vi "openUMARov.vi"() -> ()   [LabVIEW 2019]
uses:
  <userlib>/ROS for LabVIEW Software/Examples/ROS Examples/Control 1.ctl
  <userlib>/ROS for LabVIEW Software/ROS/Code/Console/Servers/ServerSubs/TopicDef.ctl
  <userlib>/ROS for LabVIEW Software/ROS/Code/SubVIs/_ROSDirection.ctl
  <vilib>/event_ctls.llb/eventvkey.ctl
  <userlib>/ROS for LabVIEW Software/ROS/MessageParsing/std_msgs/subs/parse_float32_scalar.vi
  <userlib>/ROS for LabVIEW Software/ROS/MessageBuilding/std_msgs/subs/float32Scalar.vi
panel:
  in  "Size":string(combo)="mid"
  in  "Color":string(combo)="red"
  in  "Character":string
  in  "stop":bool
  out "URL:":string="http://maps.google.com/staticmap?center=51.406200,-1.307000&zoom=18&size=570x350&maptype=hybrid&markers=51.406200,-1.307000,midpurplea&key=&path=rgb:0xFF1000,weight:5|51.406200,-1.307000|51.406200,-1.307000"
  in  "Zoom":sgl=18.0 format="%#.1g"
  out "Status service is:":sgl
  out "Status is:":sgl
  in  "Y":dbl=620.0
  in  "X":dbl=420.0
  in  "Map Format":string(combo)="hybrid"
  out "Latitude":dbl
  out "Longitude":dbl
  in  "?":refnum<k7>(container)
  out "First speed:":dbl(slide) scale=-50.0..50.0
  out "Rover height is:":sgl
  out "Position covariance [0] is:":sgl
  out "Position covariance [4] is:":sgl
  out "Position covariance [8] is:":sgl
  out "Position covariance type is:":sgl
  in  "Clear":bool
  in  "stop 2":bool
  in  "Clear 2":bool
  out "Second speed:":dbl(slide) scale=-50.0..50.0
  out "Second wheel distance (cm) is:":sgl
  out "Second wheel speed is:":T1 scale=-50.0..50.0
  out "First wheel distance (cm) is:":sgl
  out "First wheel speed is:":T1 scale=-50.0..50.0
  in  "?":bool
  out "First motor current (A) is:":sgl
  out "Second motor current (A) is:":sgl
  out "Total current (A) is:":sgl
  # "OPEN   UMA   ROV"
  # "Location"
  # "Map"
  # "GPS"
  # "Balloon"
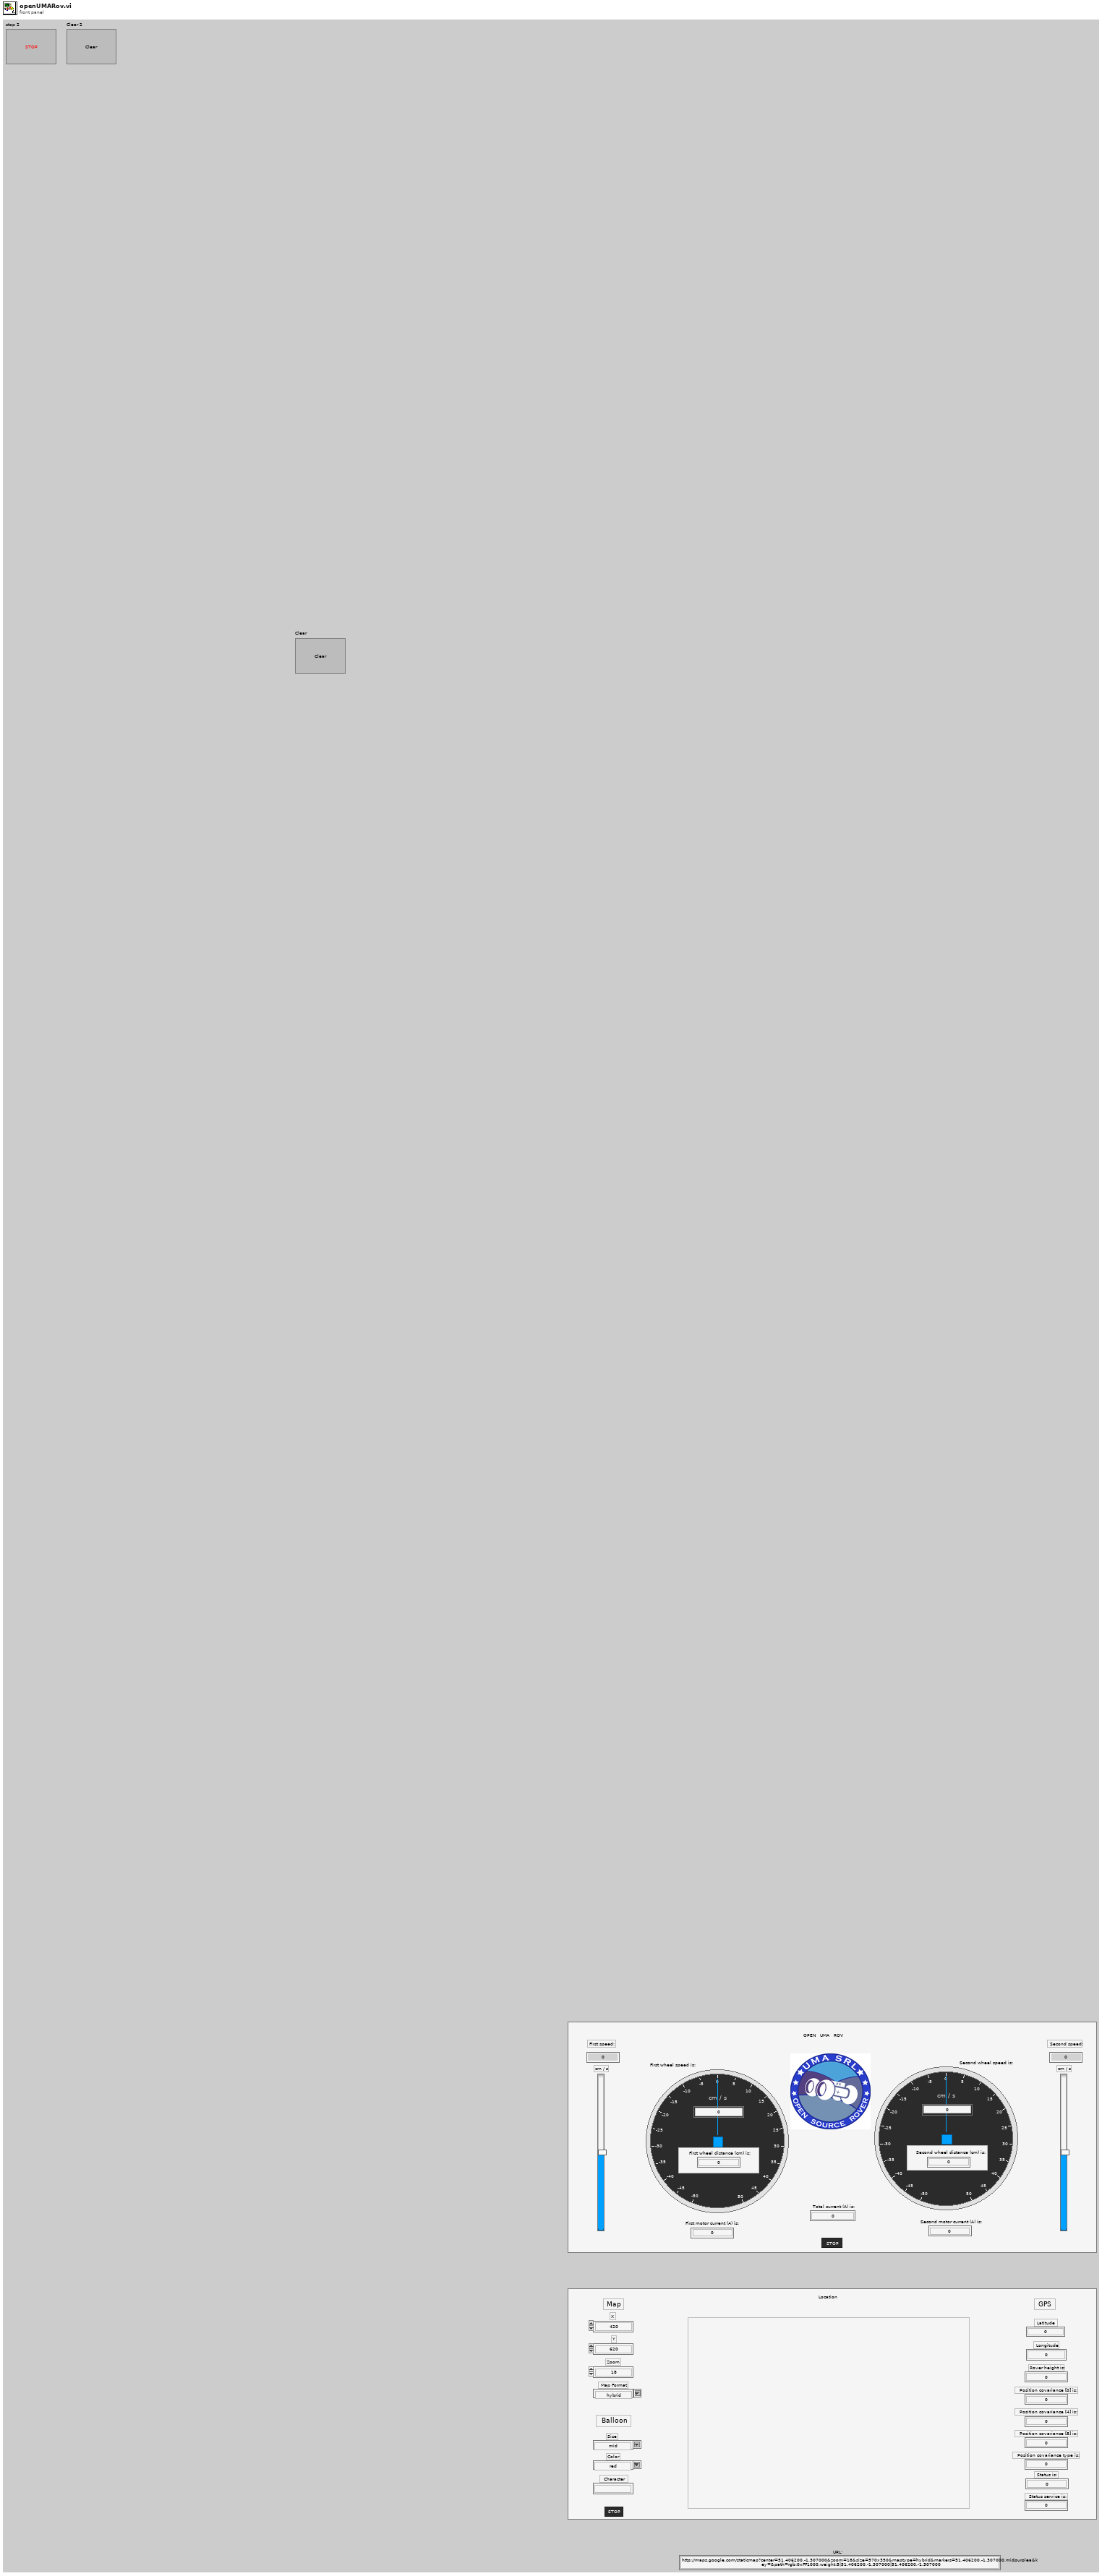
[diagram p1: front panel]
types:
  T1 = typedef "Control 1.ctl" = dbl
  T2 = typedef "TopicDef.ctl" = cluster{"Topic":string, "Type":string, "Action":T3, "Update (ms)":u16, "queue size":u16}
  T3 = typedef "_ROSDirection.ctl" = enum16{"Node", "Publisher", "Subscriber", "ServiceClient", "ServiceProvider"}
  T4 = typedef "_ROSControl.ctl" = cluster{"topic port":u16, "Node":string, "topic":string, "type":string, "node port":u16, "error ":errorcluster, "Direction":T3, "Update (ms)":u16, "FIFO size":u16}
  T5 = typedef "eventvkey.ctl" = enum16{"ASCII", "Enter", "Return", "Shift", "Ctrl", "Alt", "Cmd", "Opt", "Caps", "NumLock", "Clear", "Break", "Up", "Down", "Left", "Right", "Insert", "Delete", "Home", "End", "PageUp", "PageDown", "Escape", "Help", "Pause", "ScrollLock", "F1", "F2", "F3", "F4", "F5", "F6", "F7", "F8", "F9", "F10", "F11", "F12", "F13", "F14", "F15", "F16", "F17", "F18", "F19", "F20", "F21", "F22", "F23", "F24", "Play", "VolumeUp", "VolumeDown", "Mute", "Two Byte Char"}
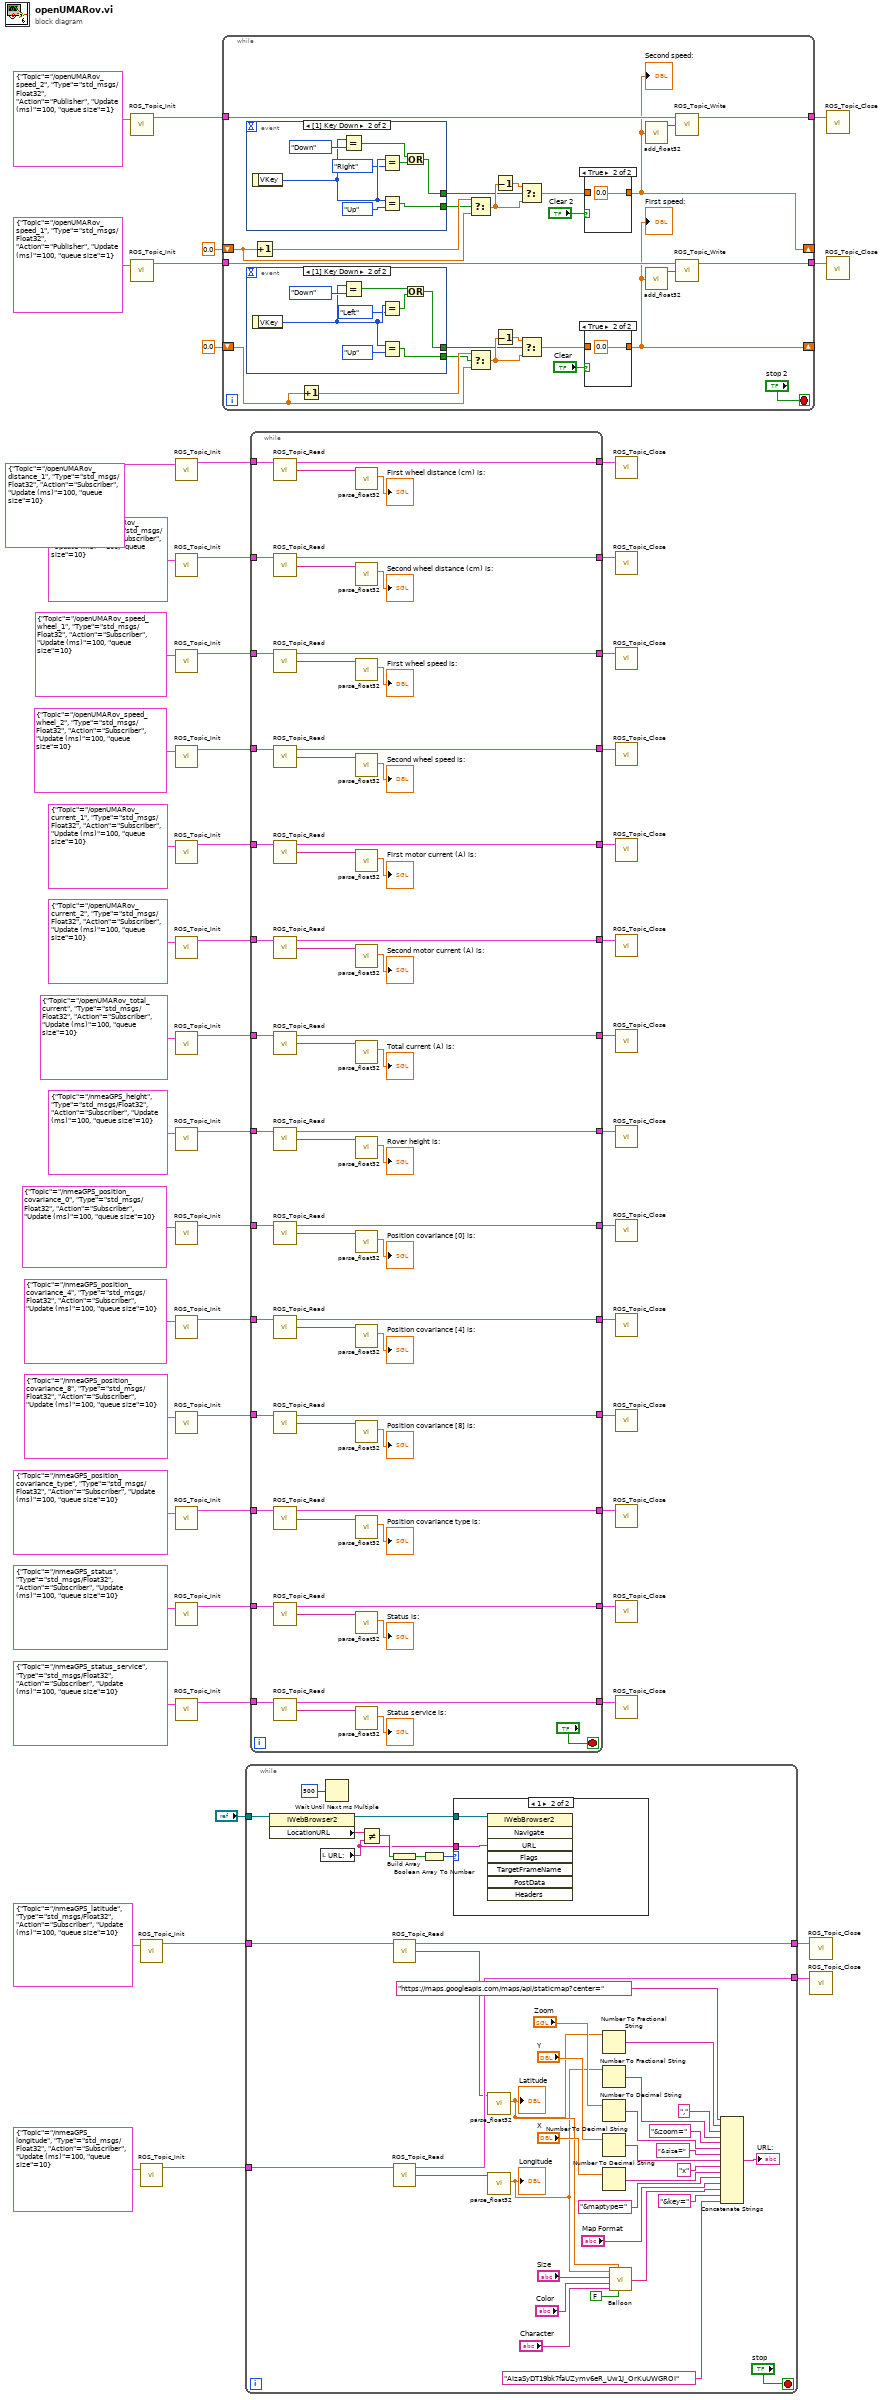
[diagram p0: block diagram]
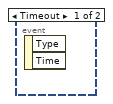
[diagram p3: hidden frame]
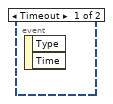
[diagram p5: hidden frame]
diagram:
  n1 = call <userlib>:"ROS_Topic_Init.vi"("Definitions"=T2 {"Topic"="/openUMARov_speed_2", "Type"="std_msgs/Float32", "Action"=enum."Publisher", "Update (ms)"=100, "queue size"=1}) -> ("ROS out"=w13:T4)  [unwired: 2 in, 1 out]
  n2 = call <userlib>:"ROS_Topic_Init.vi"("Definitions"=T2 {"Topic"="/openUMARov_speed_1", "Type"="std_msgs/Float32", "Action"=enum."Publisher", "Update (ms)"=100, "queue size"=1}) -> ("ROS out"=w10:T4)  [unwired: 2 in, 1 out]
  n3 = call <userlib>:"ROS_Topic_Init.vi"("Definitions"=T2 {"Topic"="/nmeaGPS_latitude", "Type"="std_msgs/Float32", "Action"=enum."Subscriber", "Update (ms)"=100, "queue size"=10}) -> ("ROS out"=w2:T4)  [unwired: 2 in, 1 out]
  n4 = call <userlib>:"ROS_Topic_Init.vi"("Definitions"=T2 {"Topic"="/nmeaGPS_longitude", "Type"="std_msgs/Float32", "Action"=enum."Subscriber", "Update (ms)"=100, "queue size"=10}) -> ("ROS out"=w4:T4)  [unwired: 2 in, 1 out]
  n5 = call <userlib>:"ROS_Topic_Init.vi"("Definitions"=T2 {"Topic"="/openUMARov_distance_1", "Type"="std_msgs/Float32", "Action"=enum."Subscriber", "Update (ms)"=100, "queue size"=10}) -> ("ROS out"=w56:T4)  [unwired: 2 in, 1 out]
  n6 = call <userlib>:"ROS_Topic_Init.vi"("Definitions"=T2 {"Topic"="/openUMARov_distance_2", "Type"="std_msgs/Float32", "Action"=enum."Subscriber", "Update (ms)"=100, "queue size"=10}) -> ("ROS out"=w43:T4)  [unwired: 2 in, 1 out]
  n7 = call <userlib>:"ROS_Topic_Init.vi"("Definitions"=T2 {"Topic"="/openUMARov_speed_wheel_1", "Type"="std_msgs/Float32", "Action"=enum."Subscriber", "Update (ms)"=100, "queue size"=10}) -> ("ROS out"=w41:T4)  [unwired: 2 in, 1 out]
  n8 = call <userlib>:"ROS_Topic_Init.vi"("Definitions"=T2 {"Topic"="/openUMARov_speed_wheel_2", "Type"="std_msgs/Float32", "Action"=enum."Subscriber", "Update (ms)"=100, "queue size"=10}) -> ("ROS out"=w32:T4)  [unwired: 2 in, 1 out]
  n9 = call <userlib>:"ROS_Topic_Init.vi"("Definitions"=T2 {"Topic"="/openUMARov_current_1", "Type"="std_msgs/Float32", "Action"=enum."Subscriber", "Update (ms)"=100, "queue size"=10}) -> ("ROS out"=w33:T4)  [unwired: 2 in, 1 out]
  n10 = call <userlib>:"ROS_Topic_Init.vi"("Definitions"=T2 {"Topic"="/openUMARov_current_2", "Type"="std_msgs/Float32", "Action"=enum."Subscriber", "Update (ms)"=100, "queue size"=10}) -> ("ROS out"=w34:T4)  [unwired: 2 in, 1 out]
  n11 = call <userlib>:"ROS_Topic_Init.vi"("Definitions"=T2 {"Topic"="/openUMARov_total_current", "Type"="std_msgs/Float32", "Action"=enum."Subscriber", "Update (ms)"=100, "queue size"=10}) -> ("ROS out"=w35:T4)  [unwired: 2 in, 1 out]
  n12 = call <userlib>:"ROS_Topic_Init.vi"("Definitions"=T2 {"Topic"="/nmeaGPS_height", "Type"="std_msgs/Float32", "Action"=enum."Subscriber", "Update (ms)"=100, "queue size"=10}) -> ("ROS out"=w36:T4)  [unwired: 2 in, 1 out]
  n13 = call <userlib>:"ROS_Topic_Init.vi"("Definitions"=T2 {"Topic"="/nmeaGPS_position_covariance_0", "Type"="std_msgs/Float32", "Action"=enum."Subscriber", "Update (ms)"=100, "queue size"=10}) -> ("ROS out"=w37:T4)  [unwired: 2 in, 1 out]
  n14 = call <userlib>:"ROS_Topic_Init.vi"("Definitions"=T2 {"Topic"="/nmeaGPS_position_covariance_4", "Type"="std_msgs/Float32", "Action"=enum."Subscriber", "Update (ms)"=100, "queue size"=10}) -> ("ROS out"=w38:T4)  [unwired: 2 in, 1 out]
  n15 = call <userlib>:"ROS_Topic_Init.vi"("Definitions"=T2 {"Topic"="/nmeaGPS_position_covariance_8", "Type"="std_msgs/Float32", "Action"=enum."Subscriber", "Update (ms)"=100, "queue size"=10}) -> ("ROS out"=w39:T4)  [unwired: 2 in, 1 out]
  n16 = call <userlib>:"ROS_Topic_Init.vi"("Definitions"=T2 {"Topic"="/nmeaGPS_position_covariance_type", "Type"="std_msgs/Float32", "Action"=enum."Subscriber", "Update (ms)"=100, "queue size"=10}) -> ("ROS out"=w40:T4)  [unwired: 2 in, 1 out]
  n17 = call <userlib>:"ROS_Topic_Init.vi"("Definitions"=T2 {"Topic"="/nmeaGPS_status", "Type"="std_msgs/Float32", "Action"=enum."Subscriber", "Update (ms)"=100, "queue size"=10}) -> ("ROS out"=w19:T4)  [unwired: 2 in, 1 out]
  n18 = call <userlib>:"ROS_Topic_Init.vi"("Definitions"=T2 {"Topic"="/nmeaGPS_status_service", "Type"="std_msgs/Float32", "Action"=enum."Subscriber", "Update (ms)"=100, "queue size"=10}) -> ("ROS out"=w18:T4)  [unwired: 2 in, 1 out]
  n19 = while {
    shift-right: [w71] -> _
    shift-left: 0.0 -> [w77]
    tunnel: w13 -> [w73]
    tunnel: [w72] -> w12
    tunnel: w10 -> [w61]
    tunnel: [w60] -> w9
    shift-right: [w59] -> _
    shift-left: 0.0 -> [w58]
    stop <- "stop 2" stop-if-true
    n20 = event shown="[1] Key Down" {
      selector: _ -> [_ _]
      dyn-events: _ -> [_ _]
      timeout: _ -> [_ _]
      tunnel: [_ w94] -> w75
      tunnel: [_ w93] -> w70
      event Timeout {
        n21 = event-data() -> ()  [unwired: 3 out]
      }
      event Key Down {
        n22 = event-data() -> ("VKey"=w98:T5)  [unwired: 1 out]
        n23 = Equal?(x=w98, y=eventvkey."Down") -> (x = y?=w96:bool)
        n24 = Equal?(x=w98, y=eventvkey."Right") -> (x = y?=w95:bool)
        n25 = Equal?(x=w98, y=eventvkey."Up") -> (x = y?=w93:bool)
        n26 = Or(x=w96, y=w95) -> (x .or. y?=w94:bool)
      }
    }
    n27 = event shown="[1] Key Down" {
      selector: _ -> [_ _]
      dyn-events: _ -> [_ _]
      timeout: _ -> [_ _]
      tunnel: [_ w86] -> w64
      tunnel: [_ w83] -> w62
      event Timeout {
        n28 = event-data() -> ()  [unwired: 3 out]
      }
      event Key Down {
        n29 = event-data() -> ("VKey"=w88:T5)  [unwired: 1 out]
        n30 = Equal?(x=w88, y=eventvkey."Down") -> (x = y?=w85:bool)
        n31 = Equal?(x=w88, y=eventvkey."Left") -> (x = y?=w84:bool)
        n32 = Equal?(x=w88, y=eventvkey."Up") -> (x = y?=w83:bool)
        n33 = Or(x=w85, y=w84) -> (x .or. y?=w86:bool)
      }
    }
    n34 = Increment(x=w77) -> (x+1=w80:dbl)
    n35 = Increment(x=w58) -> (x+1=w68:dbl)
    n36 = Select(t=w80, s=w70, f=w77) -> (s? t:f=w76:dbl)
    n37 = Select(t=w68, s=w62, f=w58) -> (s? t:f=w65:dbl)
    n38 = Decrement(x=w76) -> (x-1=w78:dbl)
    n39 = Decrement(x=w65) -> (x-1=w66:dbl)
    n40 = Select(t=w78, s=w75, f=w76) -> (s? t:f=w79:dbl)
    n41 = Select(t=w66, s=w64, f=w65) -> (s? t:f=w67:dbl)
    n42 = case shown="True" "Clear 2" {
      tunnel: w79 -> [w101 _]
      tunnel: [w101 0.0] -> w71
      frame False {
      }
      frame True {
      }
    }
    "Second speed:" <- w71
    n43 = case shown="True" "Clear" {
      tunnel: w67 -> [w91 _]
      tunnel: [w91 0.0] -> w59
      frame False {
      }
      frame True {
      }
    }
    "First speed:" <- w59
    n44 = call-poly <userlib>:"add_float32.vi"("Numeric"=w71) -> ("msg out"=w74:string)  [unwired: 4 in]
    n45 = call-poly <userlib>:"add_float32.vi"("Numeric"=w59) -> ("msg out"=w63:string)  [unwired: 4 in]
    n46 = call <userlib>:"ROS_Topic_Write.vi"("Msg in"=w74, "ROS in"=w73) -> ("ROS out"=w72:T4)  [unwired: 2 in, 1 out]
    n47 = call <userlib>:"ROS_Topic_Write.vi"("Msg in"=w63, "ROS in"=w61) -> ("ROS out"=w60:T4)  [unwired: 2 in, 1 out]
  }
  n48 = while {
    tunnel: "?" -> [w141]
    tunnel: w4 -> [w111]
    tunnel: [w110] -> w3
    tunnel: w2 -> [w108]
    tunnel: [w107] -> w1
    stop <- "stop" stop-if-true
    n49 = property class="IWebBrowser2"(reference=w141) -> (reference out=w140:refnum<k7>, "LocationURL"=w138:string)  [unwired: 1 in, 1 out]
    n50 = local read "URL:"() -> (w135:string)
    n51 = Wait Until Next ms Multiple(millisecond multiple=u32 500) -> ()  [unwired: 1 out]
    n52 = Not Equal?(x=w138, y=w135) -> (x != y?=w139:bool)
    n53 = Build Array(w139) -> (w137:bool[])
    n54 = call <userlib>:"ROS_Topic_Read.vi"("ROS in"=w108) -> ("Reply"=w109:string, "ROS out"=w107:T4)  [unwired: 2 in, 1 out]
    n55 = call <userlib>:"ROS_Topic_Read.vi"("ROS in"=w111) -> ("Reply"=w112:string, "ROS out"=w110:T4)  [unwired: 2 in, 1 out]
    n56 = Boolean Array To Number(Boolean array=w137) -> (number=w136:u32)
    n57 = case shown="1" w136 {
      tunnel: w135 -> [_ w144]
      tunnel: w140 -> [_ w143]
      frame 0, Default {
      }
      frame 1 {
        n58 = invoke class="IWebBrowser2" method="Navigate"(reference=w143, "URL"=w144) -> ()  [unwired: 6 in, 8 out]
      }
    }
    n59 = call-poly <userlib>:"parse_float32.vi"("msg in"=w109) -> ("number"=w106:sgl)  [unwired: 4 in, 2 out]
    "Latitude" <- w106
    n60 = call-poly <userlib>:"parse_float32.vi"("msg in"=w112) -> ("number"=w105:sgl)  [unwired: 4 in, 2 out]
    "Longitude" <- w105
    n61 = Number To Fractional String(number=w106) -> (F-format string=w116:string)  [unwired: 3 in]
    n62 = Number To Fractional String(number=w105) -> (F-format string=w115:string)  [unwired: 3 in]
    n63 = Number To Decimal String(number="Zoom") -> (decimal integer string=w130:string)  [unwired: 1 in]
    n64 = Number To Decimal String(number="Y") -> (decimal integer string=w126:string)  [unwired: 1 in]
    n65 = Number To Decimal String(number="X") -> (decimal integer string=w124:string)  [unwired: 1 in]
    n66 = call "Balloon.vi"("One more?"=FALSE, "Latitude"=w106, "Character"="Character", "Color"="Color", "Size"="Size", "Longitude"=w105) -> ("Balloon"=w121:string)
    n67 = Concatenate Strings("https://maps.googleapis.com/maps/api/staticmap?center=" ("URL"), w116, "," ("string"), w115, "&zoom=", w130, "&size=", w126, "x", w124, "&maptype=", "Map Format", w121, "&key=" ("string"), "AIzaSyDT19bk7faUZymv6eR_Uw1J_OrKuUWGROI") -> (→"URL:":string)
  }
  n68 = while {
    tunnel: w56 -> [w201]
    tunnel: [w199] -> w55
    tunnel: w43 -> [w198]
    tunnel: [w197] -> w42
    tunnel: w41 -> [w196]
    tunnel: w40 -> [w195]
    tunnel: w39 -> [w194]
    tunnel: w38 -> [w193]
    tunnel: w37 -> [w192]
    tunnel: w36 -> [w191]
    tunnel: w35 -> [w190]
    tunnel: w34 -> [w189]
    tunnel: w33 -> [w188]
    tunnel: w32 -> [w187]
    tunnel: [w186] -> w31
    tunnel: [w185] -> w30
    tunnel: [w184] -> w29
    tunnel: [w183] -> w28
    tunnel: [w182] -> w27
    tunnel: [w181] -> w26
    tunnel: [w180] -> w25
    tunnel: [w179] -> w24
    tunnel: [w178] -> w23
    tunnel: [w177] -> w22
    tunnel: w19 -> [w148]
    tunnel: w18 -> [w147]
    tunnel: [w146] -> w17
    tunnel: [w145] -> w16
    stop <- "?" stop-if-true
    n69 = call <userlib>:"ROS_Topic_Read.vi"("ROS in"=w201) -> ("Reply"=w166:string, "ROS out"=w199:T4)  [unwired: 2 in, 1 out]
    n70 = call <userlib>:"ROS_Topic_Read.vi"("ROS in"=w198) -> ("Reply"=w165:string, "ROS out"=w197:T4)  [unwired: 2 in, 1 out]
    n71 = call <userlib>:"ROS_Topic_Read.vi"("ROS in"=w196) -> ("Reply"=w164:string, "ROS out"=w186:T4)  [unwired: 2 in, 1 out]
    n72 = call <userlib>:"ROS_Topic_Read.vi"("ROS in"=w187) -> ("Reply"=w163:string, "ROS out"=w177:T4)  [unwired: 2 in, 1 out]
    n73 = call <userlib>:"ROS_Topic_Read.vi"("ROS in"=w188) -> ("Reply"=w162:string, "ROS out"=w178:T4)  [unwired: 2 in, 1 out]
    n74 = call <userlib>:"ROS_Topic_Read.vi"("ROS in"=w189) -> ("Reply"=w161:string, "ROS out"=w179:T4)  [unwired: 2 in, 1 out]
    n75 = call <userlib>:"ROS_Topic_Read.vi"("ROS in"=w190) -> ("Reply"=w160:string, "ROS out"=w180:T4)  [unwired: 2 in, 1 out]
    n76 = call <userlib>:"ROS_Topic_Read.vi"("ROS in"=w191) -> ("Reply"=w159:string, "ROS out"=w181:T4)  [unwired: 2 in, 1 out]
    n77 = call <userlib>:"ROS_Topic_Read.vi"("ROS in"=w192) -> ("Reply"=w158:string, "ROS out"=w182:T4)  [unwired: 2 in, 1 out]
    n78 = call <userlib>:"ROS_Topic_Read.vi"("ROS in"=w193) -> ("Reply"=w157:string, "ROS out"=w183:T4)  [unwired: 2 in, 1 out]
    n79 = call <userlib>:"ROS_Topic_Read.vi"("ROS in"=w194) -> ("Reply"=w156:string, "ROS out"=w184:T4)  [unwired: 2 in, 1 out]
    n80 = call <userlib>:"ROS_Topic_Read.vi"("ROS in"=w195) -> ("Reply"=w155:string, "ROS out"=w185:T4)  [unwired: 2 in, 1 out]
    n81 = call <userlib>:"ROS_Topic_Read.vi"("ROS in"=w148) -> ("Reply"=w152:string, "ROS out"=w145:T4)  [unwired: 2 in, 1 out]
    n82 = call <userlib>:"ROS_Topic_Read.vi"("ROS in"=w147) -> ("Reply"=w149:string, "ROS out"=w146:T4)  [unwired: 2 in, 1 out]
    n83 = call-poly <userlib>:"parse_float32.vi"("msg in"=w166) -> ("number"=→"First wheel distance (cm) is:":sgl)  [unwired: 4 in, 2 out]
    n84 = call-poly <userlib>:"parse_float32.vi"("msg in"=w165) -> ("number"=→"Second wheel distance (cm) is:":sgl)  [unwired: 4 in, 2 out]
    n85 = call-poly <userlib>:"parse_float32.vi"("msg in"=w164) -> ("number"=→"First wheel speed is:":sgl)  [unwired: 4 in, 2 out]
    n86 = call-poly <userlib>:"parse_float32.vi"("msg in"=w163) -> ("number"=→"Second wheel speed is:":sgl)  [unwired: 4 in, 2 out]
    n87 = call-poly <userlib>:"parse_float32.vi"("msg in"=w162) -> ("number"=→"First motor current (A) is:":sgl)  [unwired: 4 in, 2 out]
    n88 = call-poly <userlib>:"parse_float32.vi"("msg in"=w161) -> ("number"=→"Second motor current (A) is:":sgl)  [unwired: 4 in, 2 out]
    n89 = call-poly <userlib>:"parse_float32.vi"("msg in"=w160) -> ("number"=→"Total current (A) is:":sgl)  [unwired: 4 in, 2 out]
    n90 = call-poly <userlib>:"parse_float32.vi"("msg in"=w159) -> ("number"=→"Rover height is:":sgl)  [unwired: 4 in, 2 out]
    n91 = call-poly <userlib>:"parse_float32.vi"("msg in"=w158) -> ("number"=→"Position covariance [0] is:":sgl)  [unwired: 4 in, 2 out]
    n92 = call-poly <userlib>:"parse_float32.vi"("msg in"=w157) -> ("number"=→"Position covariance [4] is:":sgl)  [unwired: 4 in, 2 out]
    n93 = call-poly <userlib>:"parse_float32.vi"("msg in"=w156) -> ("number"=→"Position covariance [8] is:":sgl)  [unwired: 4 in, 2 out]
    n94 = call-poly <userlib>:"parse_float32.vi"("msg in"=w155) -> ("number"=→"Position covariance type is:":sgl)  [unwired: 4 in, 2 out]
    n95 = call-poly <userlib>:"parse_float32.vi"("msg in"=w152) -> ("number"=→"Status is:":sgl)  [unwired: 4 in, 2 out]
    n96 = call-poly <userlib>:"parse_float32.vi"("msg in"=w149) -> ("number"=→"Status service is:":sgl)  [unwired: 4 in, 2 out]
  }
  n97 = call <userlib>:"ROS_Topic_Close.vi"("ROS in"=w55) -> ()  [unwired: 3 in, 1 out]
  n98 = call <userlib>:"ROS_Topic_Close.vi"("ROS in"=w42) -> ()  [unwired: 3 in, 1 out]
  n99 = call <userlib>:"ROS_Topic_Close.vi"("ROS in"=w31) -> ()  [unwired: 3 in, 1 out]
  n100 = call <userlib>:"ROS_Topic_Close.vi"("ROS in"=w22) -> ()  [unwired: 3 in, 1 out]
  n101 = call <userlib>:"ROS_Topic_Close.vi"("ROS in"=w23) -> ()  [unwired: 3 in, 1 out]
  n102 = call <userlib>:"ROS_Topic_Close.vi"("ROS in"=w24) -> ()  [unwired: 3 in, 1 out]
  n103 = call <userlib>:"ROS_Topic_Close.vi"("ROS in"=w25) -> ()  [unwired: 3 in, 1 out]
  n104 = call <userlib>:"ROS_Topic_Close.vi"("ROS in"=w26) -> ()  [unwired: 3 in, 1 out]
  n105 = call <userlib>:"ROS_Topic_Close.vi"("ROS in"=w27) -> ()  [unwired: 3 in, 1 out]
  n106 = call <userlib>:"ROS_Topic_Close.vi"("ROS in"=w28) -> ()  [unwired: 3 in, 1 out]
  n107 = call <userlib>:"ROS_Topic_Close.vi"("ROS in"=w29) -> ()  [unwired: 3 in, 1 out]
  n108 = call <userlib>:"ROS_Topic_Close.vi"("ROS in"=w30) -> ()  [unwired: 3 in, 1 out]
  n109 = call <userlib>:"ROS_Topic_Close.vi"("ROS in"=w16) -> ()  [unwired: 3 in, 1 out]
  n110 = call <userlib>:"ROS_Topic_Close.vi"("ROS in"=w17) -> ()  [unwired: 3 in, 1 out]
  n111 = call <userlib>:"ROS_Topic_Close.vi"("ROS in"=w1) -> ()  [unwired: 3 in, 1 out]
  n112 = call <userlib>:"ROS_Topic_Close.vi"("ROS in"=w3) -> ()  [unwired: 3 in, 1 out]
  n113 = call <userlib>:"ROS_Topic_Close.vi"("ROS in"=w12) -> ()  [unwired: 3 in, 1 out]
  n114 = call <userlib>:"ROS_Topic_Close.vi"("ROS in"=w9) -> ()  [unwired: 3 in, 1 out]
